vi "Convert DPID Name String to DPID ID.vi"(11 "DPID Name":string) -> (3 "DPID ID":u8)   [LabVIEW 2015, in "Diagnostics Addon Shared.lvlib"]
uses:
  Diagnostics Addon Shared.lvlib
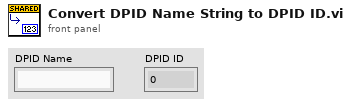
[diagram p1: front panel]
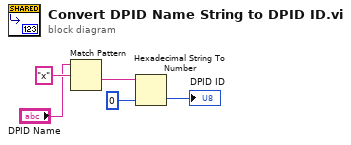
[diagram p0: block diagram]
diagram:
  n1 = Match Pattern(string="DPID Name", regular expression="x") -> (after substring=w3:string)  [unwired: 1 in, 3 out]
  n2 = Hexadecimal String To Number(string=w3, default (0uL)=u8 0 ("default (0 U32)")) -> (number=→"DPID ID":u8)  [unwired: 1 in, 1 out]
